vi "Filter by Device Address.vi"(0 "CAN Frame":T1 {"payload" format="%x"; "timestamp" format="%<%.7X\n%x>T"; "type" items=["CAN Data"=0, "CAN Remote"=1, "CAN Bus Error"=2, "Delay"=224, "Log Trigger"=225, "Start Trigger"=226]; "identifier" format="%x"}, 7 "Current Device Address":u8, 11 "error in":errorcluster) -> (8 "Pass Through":bool, 15 "error out":errorcluster)   [LabVIEW 2013, in "J1939 Utilities.lvlib"]
uses:
  J1939 Utilities.lvlib
  <vilib>/xnet/xnet.llb/XNET Frame CAN.ctl
  <vilib>/xnet/xnet.llb/XNET Frame Type CAN.ctl
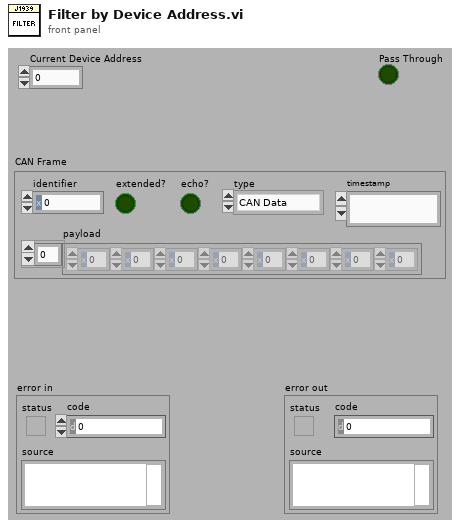
[diagram p1: front panel]
types:
  T1 = typedef "XNET Frame CAN.ctl" = cluster{"timestamp":timestamp, "payload":u8[], "identifier":u32, "type":T2, "extended?":bool, "echo?":bool}
  T2 = typedef "XNET Frame Type CAN.ctl" = u8
  T3 = typedef "J1939 Utilities.lvlib/Message Types.ctl" = enum8{"PDU 1", "RQST2", "XFER", "ACKM", "RQST", "TP.DT - RTS/CTS", "TP.DT - BAM", "TP.CM - RTS", "TP.CM - CTS", "TP.CM - EndofMsgACK", "TP.CM - BAM", "TP.CM - Abort", "TP.CM - Error", "ACL", "Proprietary A", "PDU 2", "Proprietary B", "Error"}
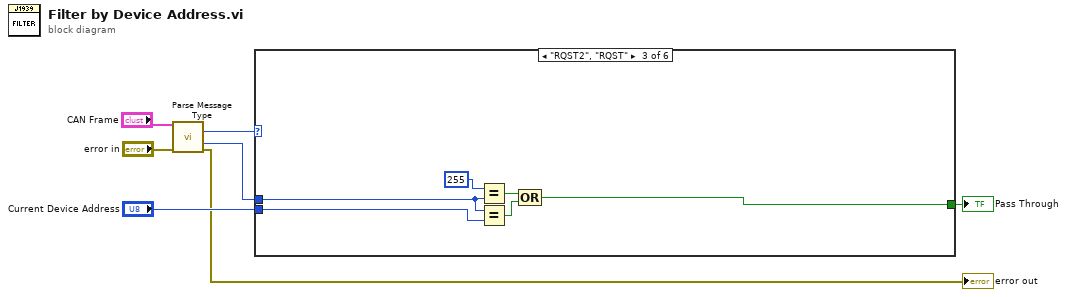
[diagram p0: block diagram]
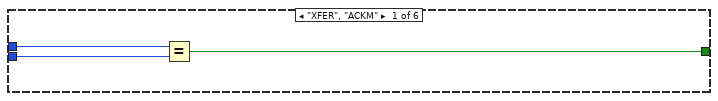
[diagram p2: hidden frame]
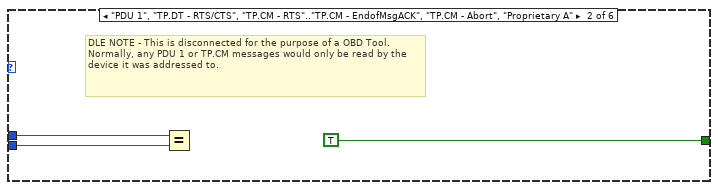
[diagram p3: hidden frame]
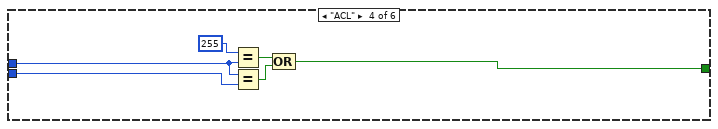
[diagram p4: hidden frame]
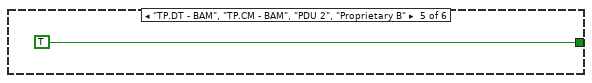
[diagram p5: hidden frame]
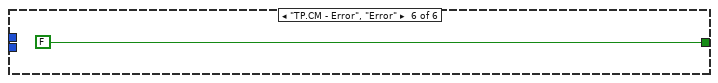
[diagram p6: hidden frame]
diagram:
  n1 = call "Parse Message Type.vi"("CAN frame"="CAN Frame", "error in"="error in") -> ("State"=w7:T3, "PDU S"=w6:u8, "error out"=→"error out":errorcluster)  [unwired: 11 out]
  n2 = case shown="\"RQST2\", \"RQST\"" w7 {
    tunnel: "Current Device Address" -> [w10 w13 w16 w22 _ _]
    tunnel: w6 -> [w9 w12 w14 w20 _ _]
    tunnel: [w8 TRUE w15 w21 TRUE FALSE] -> w4
    frame "XFER", "ACKM" {
      n3 = Equal?(x=w9, y=w10) -> (x = y?=w8:bool)
    }
    frame "PDU 1", "TP.DT - RTS/CTS", "TP.CM - RTS".."TP.CM - EndofMsgACK", "TP.CM - Abort", "Proprietary A" {
      # "DLE NOTE - This is disconnected for the purpose of a OBD Tool.  Normally, any PDU 1 or TP.CM messages would only be read by the device it was addressed to."
      n4 = Equal?(x=w12, y=w13) -> ()  [unwired: 1 out]
    }
    frame "RQST2", "RQST" {
      n5 = Equal?(x=u8 255 ("y"), y=w14) -> (x = y?=w17:bool)
      n6 = Equal?(x=w14, y=w16) -> (x = y?=w18:bool)
      n7 = Compound Arithmetic op=OR(w17, w18) -> (w15:bool)
    }
    frame "ACL" {
      n8 = Equal?(x=u8 255 ("y"), y=w20) -> (x = y?=w23:bool)
      n9 = Equal?(x=w20, y=w22) -> (x = y?=w24:bool)
      n10 = Compound Arithmetic op=OR(w23, w24) -> (w21:bool)
    }
    frame "TP.DT - BAM", "TP.CM - BAM", "PDU 2", "Proprietary B" {
    }
    frame "TP.CM - Error", "Error" {
    }
  }
  "Pass Through" <- w4
